vi "CANOpen_Main_Cleanup FIFOs.vi"(11 "Data":T25 {"CD Settings"."Status NMT"."Hardware Output"."Channel Pairs"."Chan Refs"."Data Reference" format="%.0x"; "CD Settings"."Status NMT"."Hardware Input"."Channel Pairs"."Chan Refs" format="%.0x"; "CD Settings"."SDO Asynch"."HW Dyn Read"."Resp Chan."."Chan Refs" format="%.0x"; "CD Settings"."SDO Asynch"."HW Dyn Read"."Req Chan."."Chan Refs" format="%.0x"; "CD Settings"."SDO Asynch"."HW Dyn Write"."Resp Chan."."Chan Refs" format="%.0x"; "CD Settings"."SDO Asynch"."HW Dyn Write"."Req Chan."."Chan Refs" format="%.0x"; "CD Settings"."SDO Asynch"."List SDO"."Resp Chan."."Chan Refs" format="%.0x"; "CD Settings"."SDO Asynch"."List SDO"."Req Chan."."Chan Refs" format="%.0x"; "CD Settings"."Bus Commands"."Hardware Output"."Channel Pairs"."Chan Refs" format="%.0x"; "CD Settings"."Data References"."Hardware Input"."Channel Pairs"."Chan Refs" format="%.0x"; "CD Settings"."Data References"."Hardware Output"."Channel Pairs"."Block Refs"."Data Reference" format="%.0x"; "CD Settings"."Driver Settings"."CANOpen Bus Settings"."Baud Rate" items=["1 Mbit/s"=0, "800 kbit/s"=1, "500 kbit/s"=2, "250 kbit/s"=3, "125 kbit/s"=4, "50 kbit/s"=6, "20 kbit/s"=7, "10 kbit/s"=8]; "CD Settings"."Driver Settings"."CANOpen Bus Settings"."CANOpen Interface Name" items=["CANopen01", "CANopen02", "CANopen03", "CANopen04", "CANopen05", "CANopen06", "CANopen07", "CANopen08", "CANopen09", "CANopen10", "CANopen11", "CANopen12", "CANopen13", "CANopen14", "CANopen15", "CANopen16", "CANopen17", "CANopen18", "CANopen19", "CANopen20", "CANopen21", "CANopen22", "CANopen23", "CANopen24", "CANopen25", "CANopen26", "CANopen27", "CANopen28", "CANopen29", "CANopen30", "CANopen31", "CANopen32"]; "CD Settings"."Driver Settings"."Nodes"."NMT"."Node init static SDO state" items=["start remote node"=1, "enter pre-operational"=128]; "CD Settings"."Driver Settings"."Nodes"."NMT"."Node run state" items=["start remote node"=1, "stop remote node"=2, "enter pre-operational"=128, "reset node"=129, "reset communication"=130]; "CD Settings"."Driver Settings"."Nodes"."Dynamic SDOs"."Block Data" format="%.0x"; "CD Settings"."Driver Settings"."Nodes"."RPDOs"."PDO Channel" items=["PDO 1", "PDO 2", "PDO 3", "PDO 4"]; "CD Settings"."Driver Settings"."Nodes"."TPDOs"."PDO Channel" items=["PDO 1", "PDO 2", "PDO 3", "PDO 4"]; "CD Settings"."Driver Settings"."Nodes"."SDOs"."Block Data" format="%.0x"}) -> (0 "error out":errorcluster)   [LabVIEW 2013, in "CANOpen Addon Custom Device.lvlib"]
uses:
  CANOpen Addon Custom Device.lvlib
  SubVIS/Error Handling API/_Controls/VS Errors_Error Handling Cluster.ctl
  SubVIS/CANOpen_Settings.ctl
  SubVIS/CANOpen_Node Settings.ctl
  Shared Code/CANOpen_Bus Settings.ctl
  Shared Code/CANOpen Interface Name.ctl
  <vilib>/CANopenLib/CANOPEN.llb/CANopen BaudRate.ctl
  SubVIS/CANOpen_Node Message Settings.ctl
  Shared Code/CANOpen_PDO Settings.ctl
  Shared Code/CANOpen_PDO Parameter Settings.ctl
  Shared Code/CANOpen_PDO Data Type.ctl
  System Explorer/SubVIs/CANopen Byte Order.ctl
  Shared Code/CANOpen_SDO Settings.ctl
  SubVIS/CANOpen_NMT Settings.ctl
  CanOpen_NMT_Config.ctl
  CanOpen_NMT_Static detect.ctl
  CanOpen_Main Node Ids.ctl
  SubVIS/CANOpen_VS Data Refs.ctl
  <vilib>/NI Veristand/Custom Device API/Data Reference.ctl
  <vilib>/NI Veristand/Custom Device API/Block Data Reference.ctl
  SubVIS/CANOpen_VS Bidirectional Data Refs.ctl
  SubVIS/CANOpen_VS SDOs Data Refs.ctl
  CanOpen_SDO Dynamic queue.ctl
  Shared Code/CANOpen_SDO queue W data.ctl
  Shared Code/CANOpen_SDO queue mode.ctl
  Shared Code/CANOpen_PDO Data Type in queue.ctl
  SubVIS/CANOpen_VS Status Management Data Refs.ctl
  CanOpen_NMT_HWOut_ChannelPairs.ctl
  CanOpen_NMT_HWIn_ChannelPairs.ctl
  <vilib>/NI Veristand/Custom Device API/Custom Device API.lvlib
panel:
  # "LSB"
  # "MSB"
  # "LSB"
  # "MSB"
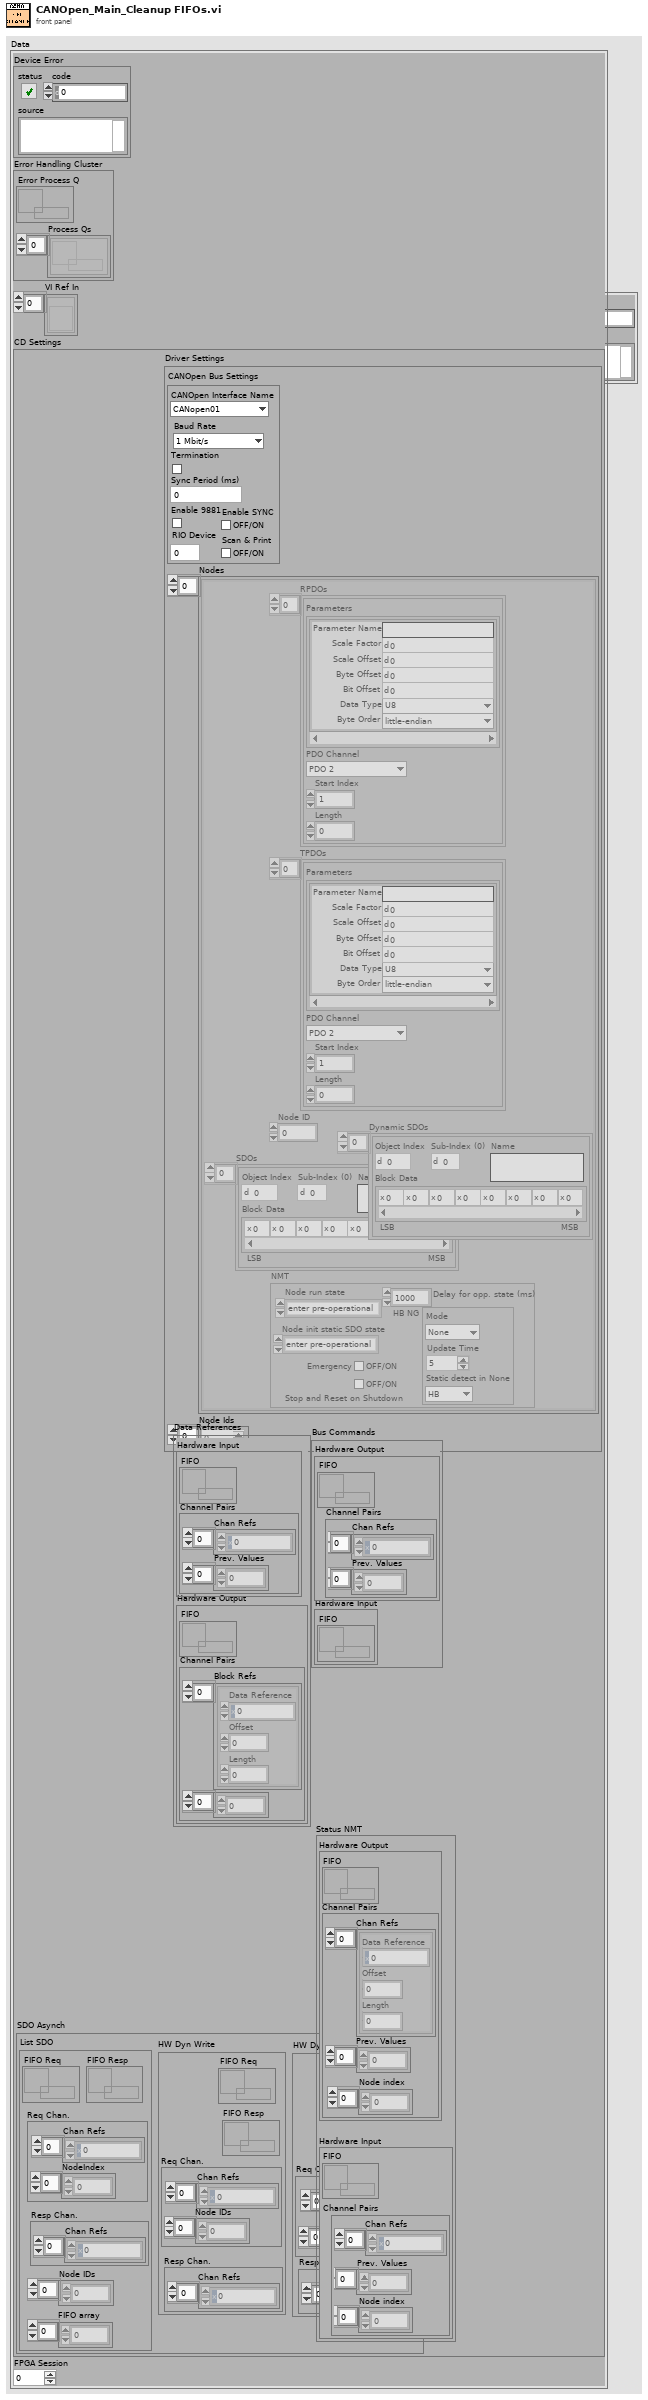
[diagram p1: front panel]
types:
  T1 = typedef "CANOpen Addon Custom Device.lvlib/VS Errors_Error Handling Cluster.ctl" = cluster{"Error Process Q":refnum<queue>, "Process Qs":refnum<queue>[]}
  T2 = typedef "CANOpen_Settings.ctl" = cluster{"Driver Settings":T3, "Data References":T17, "Bus Commands":T20, "SDO Asynch":T21, "Status NMT":T22}
  T3 = typedef "CANOpen_Node Settings.ctl" = cluster{"CANOpen Bus Settings":T4, "Nodes":T7[], "Node Ids":T16}
  T4 = typedef "CANOpen Addon Custom Device.lvlib/CANOpen_Bus Settings.ctl" = cluster{"CANOpen Interface Name":T5, "Baud Rate":T6, "Termination":bool, "Sync Period (ms)":i64, "Enable 9881":bool, "RIO Device":u16, "Enable SYNC":bool, "Scan & Print":bool}
  T5 = typedef "CANOpen Addon Custom Device.lvlib/CANOpen Interface Name.ctl" = u32
  T6 = typedef "CANopen BaudRate.ctl" = u32
  T7 = typedef "CANOpen_Node Message Settings.ctl" = cluster{"RPDOs":T8[], "TPDOs":T8[], "Node ID":u8, "SDOs":T12[], "Dynamic SDOs":T12[], "NMT":T13}
  T8 = typedef "CANOpen Addon Custom Device.lvlib/CANOpen_PDO Settings.ctl" = cluster{"Parameters":T9[], "PDO Channel":u8, "Start Index":u32, "Length":u32}
  T9 = typedef "CANOpen Addon Custom Device.lvlib/CANOpen_PDO Parameter Settings.ctl" = cluster{"Parameter Name":string, "Scale Factor":dbl, "Scale Offset":dbl, "Byte Offset":u8, "Bit Offset":u8, "Data Type":T10, "Byte Order":T11}
  T10 = typedef "CANOpen Addon Custom Device.lvlib/CANOpen_PDO Data Type.ctl" = enum16{"U8", "U16", "U32", "I8", "I16", "I32", "Single", "Double", "Boolean"}
  T11 = typedef "CANOpen Addon Custom Device.lvlib/CANopen Byte Order.ctl" = enum16{"big-endian network order", "little-endian"}
  T12 = typedef "CANOpen Addon Custom Device.lvlib/CANOpen_SDO Settings.ctl" = cluster{"Object Index":u16, "Sub-Index (0)":u8, "Block Data":u8[], "Name":string}
  T13 = typedef "CANOpen Addon Custom Device.lvlib/CANOpen_NMT Settings.ctl" = cluster{"Node run state":u16, "Emergency":bool, "HB NG":T14, "Delay for opp. state (ms)":dbl, "Node init static SDO state":u16, "Stop and Reset on Shutdown":bool}
  T14 = typedef "CANOpen Addon Custom Device.lvlib/CanOpen_NMT_Config.ctl" = cluster{"Mode":T15, "Update Time":u16, "Static detect in None":T15}
  T15 = typedef "CANOpen Addon Custom Device.lvlib/CanOpen_NMT_Static detect.ctl" = enum16{"None", "HB", "NG"}
  T16 = typedef "CANOpen Addon Custom Device.lvlib/CanOpen_Main Node Ids.ctl" = u8[]
  T17 = typedef "CANOpen_VS Data Refs.ctl" = cluster{"Hardware Input":cluster{"FIFO":refnum<k33>, "Channel Pairs":cluster{"Chan Refs":T18[], "Prev. Values":dbl[]}}, "Hardware Output":cluster{"FIFO":refnum<k33>, "Channel Pairs":cluster{"Block Refs":T19[], "Prev. Values":dbl[]}}}
  T18 = typedef "Custom Device API.lvlib/Data Reference.ctl" = i32
  T19 = typedef "Custom Device API.lvlib/Block Data Reference.ctl" = cluster{"Data Reference":T18, "Offset":i32, "Length":i32}
  T20 = typedef "CANOpen_VS Bidirectional Data Refs.ctl" = cluster{"Hardware Output":cluster{"FIFO":refnum<k33>, "Channel Pairs":cluster{"Chan Refs":T18[], "Prev. Values":dbl[]}}, "Hardware Input":cluster{"FIFO":refnum<k33>}}
  T21 = typedef "CANOpen Addon Custom Device.lvlib/CANOpen_VS SDOs Data Refs.ctl" = cluster{"List SDO":cluster{"FIFO Req":refnum<k33>, "Req Chan.":cluster{"Chan Refs":T18[], "NodeIndex":dbl[]}, "FIFO Resp":refnum<k33>, "Resp Chan.":cluster{"Chan Refs":T18[]}, "Node IDs":u8[], "FIFO array":dbl[]}, "HW Dyn Write":cluster{"FIFO Req":refnum<k33>, "FIFO Resp":refnum<k33>, "Req Chan.":cluster{"Chan Refs":T18[], "Node IDs":u8[]}, "Resp Chan.":cluster{"Chan Refs":T18[]}}, "HW Dyn Read":cluster{"FIFO Req":refnum<k33>, "FIFO Resp":refnum<k33>, "Req Chan.":cluster{"Chan Refs":T18[], "Node IDs":u8[]}, "Resp Chan.":cluster{"Chan Refs":T18[]}}}
  T22 = typedef "CANOpen Addon Custom Device.lvlib/CANOpen_VS Status Management Data Refs.ctl" = cluster{"Hardware Output":cluster{"FIFO":refnum<k33>, "Channel Pairs":T23}, "Hardware Input":cluster{"FIFO":refnum<k33>, "Channel Pairs":T24}}
  T23 = typedef "CANOpen Addon Custom Device.lvlib/CanOpen_NMT_HWOut_ChannelPairs.ctl" = cluster{"Chan Refs":T19[], "Prev. Values":dbl[], "Node index":dbl[]}
  T24 = typedef "CANOpen Addon Custom Device.lvlib/CanOpen_NMT_HWIn_ChannelPairs.ctl" = cluster{"Chan Refs":T18[], "Prev. Values":dbl[], "Node index":dbl[]}
  T25 = cluster{"Device Error":errorcluster, "Error Handling Cluster":T1, "VI Ref In":refnum<vi>[], "CD Settings":T2, "FPGA Session":u32}
  T26 = cluster{"FIFO Req":refnum<k33>, "Req Chan.":cluster{"Chan Refs":T18[], "NodeIndex":dbl[]}, "FIFO Resp":refnum<k33>, "Resp Chan.":cluster{"Chan Refs":T18[]}, "Node IDs":u8[], "FIFO array":dbl[]}
  T27 = cluster{"FIFO Req":refnum<k33>, "FIFO Resp":refnum<k33>, "Req Chan.":cluster{"Chan Refs":T18[], "Node IDs":u8[]}, "Resp Chan.":cluster{"Chan Refs":T18[]}}
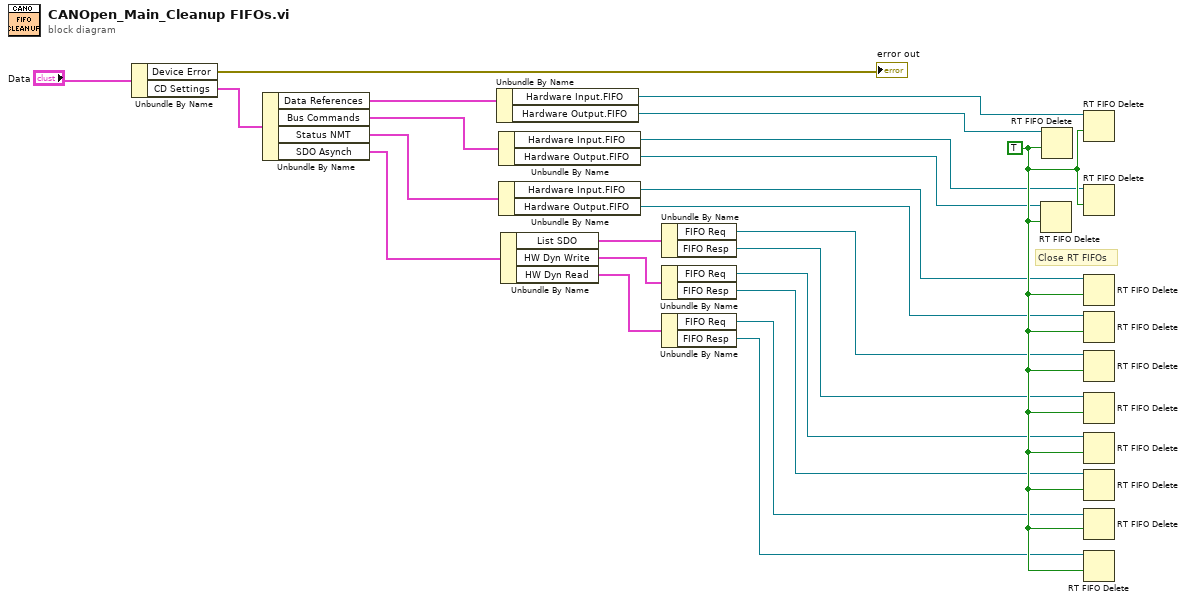
[diagram p0: block diagram]
diagram:
  w23 = TRUE
  # "Close RT FIFOs"
  n1 = Unbundle By Name("Data") -> ("Device Error"=→"error out":errorcluster, "CD Settings"=w20:T2)
  n2 = Unbundle By Name(w20) -> ("Data References"=w19:T17, "Bus Commands"=w18:T20, "Status NMT"=w17:T22, "SDO Asynch"=w10:T21)
  n3 = Unbundle By Name(w19) -> ("Hardware Input.FIFO"=w16:refnum<k33>, "Hardware Output.FIFO"=w15:refnum<k33>)
  n4 = Unbundle By Name(w18) -> ("Hardware Input.FIFO"=w14:refnum<k33>, "Hardware Output.FIFO"=w13:refnum<k33>)
  n5 = Unbundle By Name(w17) -> ("Hardware Input.FIFO"=w12:refnum<k33>, "Hardware Output.FIFO"=w11:refnum<k33>)
  n6 = Unbundle By Name(w10) -> ("List SDO"=w9:T26, "HW Dyn Write"=w8:T27, "HW Dyn Read"=w7:T27)
  n7 = Unbundle By Name(w9) -> ("FIFO Req"=w1:refnum<k33>, "FIFO Resp"=w2:refnum<k33>)
  n8 = Unbundle By Name(w8) -> ("FIFO Req"=w3:refnum<k33>, "FIFO Resp"=w4:refnum<k33>)
  n9 = Unbundle By Name(w7) -> ("FIFO Req"=w5:refnum<k33>, "FIFO Resp"=w6:refnum<k33>)
  n10 = RT FIFO Delete(0:w13, 2:w23) -> ()  [unwired: 1 in, 1 out]
  n11 = RT FIFO Delete(0:w15, 2:w23) -> ()  [unwired: 1 in, 1 out]
  n12 = RT FIFO Delete(0:w16, 2:w23) -> ()  [unwired: 1 in, 1 out]
  n13 = RT FIFO Delete(0:w14, 2:w23) -> ()  [unwired: 1 in, 1 out]
  n14 = RT FIFO Delete(0:w12, 2:w23) -> ()  [unwired: 1 in, 1 out]
  n15 = RT FIFO Delete(0:w11, 2:w23) -> ()  [unwired: 1 in, 1 out]
  n16 = RT FIFO Delete(0:w1, 2:w23) -> ()  [unwired: 1 in, 1 out]
  n17 = RT FIFO Delete(0:w2, 2:w23) -> ()  [unwired: 1 in, 1 out]
  n18 = RT FIFO Delete(0:w3, 2:w23) -> ()  [unwired: 1 in, 1 out]
  n19 = RT FIFO Delete(0:w4, 2:w23) -> ()  [unwired: 1 in, 1 out]
  n20 = RT FIFO Delete(0:w5, 2:w23) -> ()  [unwired: 1 in, 1 out]
  n21 = RT FIFO Delete(0:w6, 2:w23) -> ()  [unwired: 1 in, 1 out]
